vi "setTransactionCategory.vi"(8 "error in (no error)":errorcluster, 9 "Transaction":refnum<class "Transaction.lvclass">, 10 "Category.lvclass":refnum<class "Category.lvclass">, 11 "Database in":refnum<class "Account History.lvclass">) -> (0 "error out":errorcluster, 3 "Database out":refnum<class "Account History.lvclass">)   [LabVIEW 2018, in "Account History.lvclass"]
uses:
  Account History.lvclass
  Category/Category.lvclass
  Transaction/Transaction.lvclass
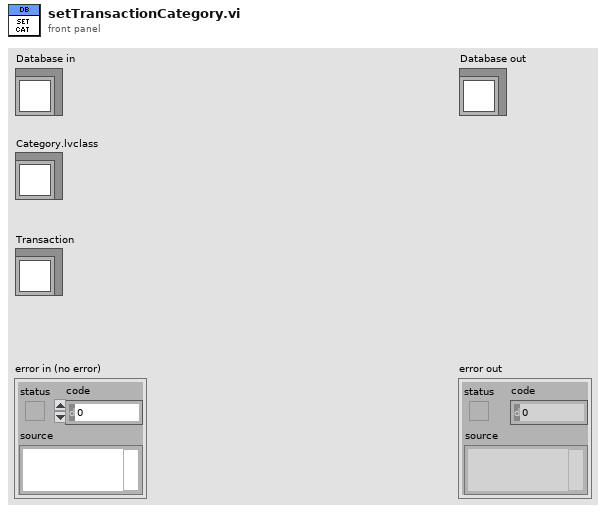
[diagram p1: front panel]
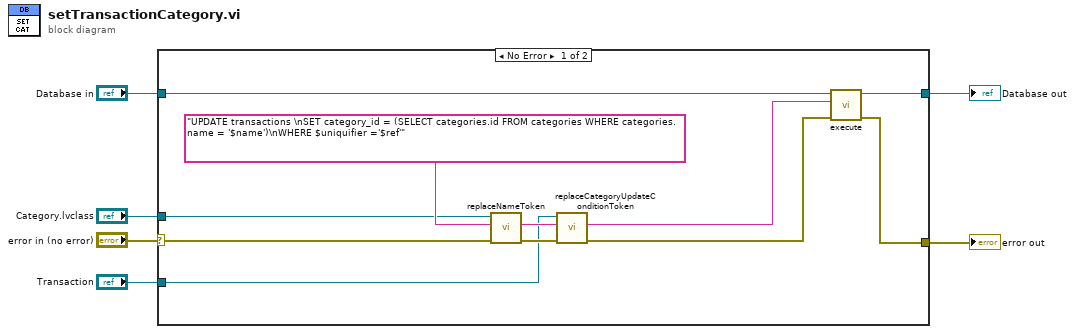
[diagram p0: block diagram]
diagram:
  n1 = case shown="No Error" "error in (no error)" {
    selector: "error in (no error)" -> [w12 w19]
    tunnel: [w15 w19] -> w5
    tunnel: [w17 w18] -> w3
    tunnel: "Database in" -> [w16 w18]
    tunnel: "Transaction" -> [w9 _]
    tunnel: "Category.lvclass" -> [w13 _]
    frame No Error {
      n2 = call "replaceNameToken.vi"("error in (no error)"=w12, "Query In"="UPDATE transactions \nSET category_id = (SELECT categories.id FROM categories WHERE categories.name = '$name')\nWHERE $uniquifier ='$ref'", "Category in"=w13) -> ("error out"=w10:errorcluster, "Query Out"=w11:string)  [unwired: 6 in, 1 out]
      n3 = call-dynamic "replaceCategoryUpdateConditionToken.vi"("error in (no error)"=w10, "Query In"=w11, "Transaction in"=w9) -> ("error out"=w8:errorcluster, "Query Out"=w7:string)  [unwired: 6 in, 1 out]
      n4 = call "execute.vi"("error in (no error)"=w8, "SQL query"=w7, "Database in"=w16) -> ("error out"=w15:errorcluster, "Database out"=w17:refnum<class "Account History.lvclass">)  [unwired: 7 in]
    }
    frame Error {
    }
  }
  "error out" <- w5
  "Database out" <- w3
